vi "CalculateCircle.vi"(5 "Robot":dbl[](array[numeric]), 6 "RealCamera":cluster{"X":dbl, "Y":dbl} {"X" format="%#_13g"}, 7 "Camera":dbl[](array[numeric]), 8 "错误输入（无错误）":errorcluster, 10 "Circle.Steps":dbl[][](array[numeric]), 11 "Circle.Points":dbl[][](array[numeric])) -> (0 "错误输出":errorcluster, 2 "RobotY":dbl, 3 "RobotX":dbl)   [LabVIEW 2016]
uses:
  X86/halcondotnet.dll
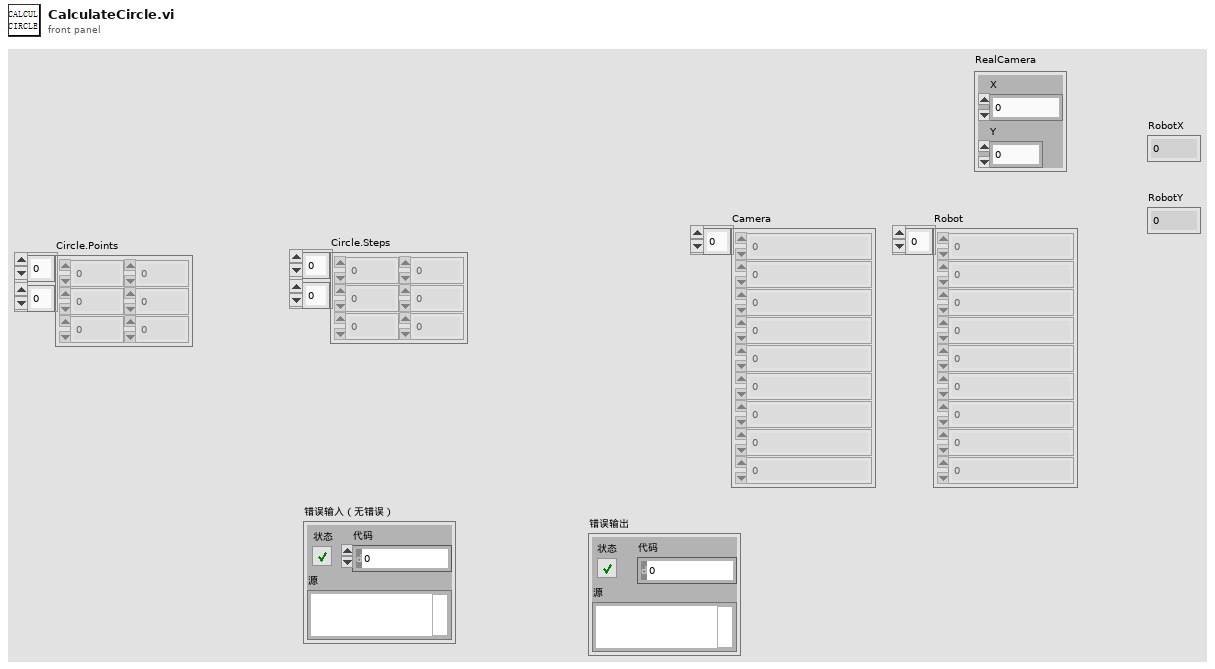
[diagram p1: front panel]
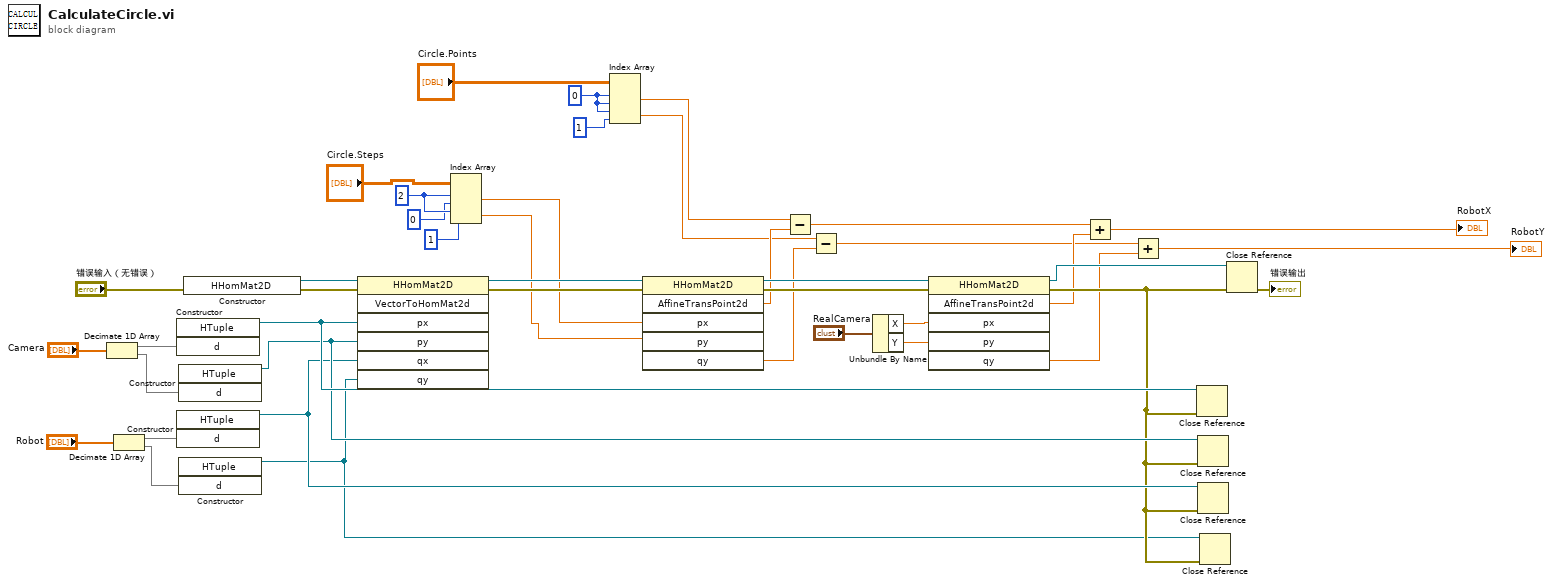
[diagram p0: block diagram]
diagram:
  w4 = 0 ("索引 (行)")
  w11 = 2 ("索引 (行)")
  n1 = Decimate 1D Array("Camera") -> (w40:dbl[], w39:dbl[])
  n2 = Decimate 1D Array("Robot") -> (w38:dbl[], w37:dbl[])
  n3 = constructor class="HTuple"("d"=w40) -> (reference out=w30:refnum<k24>)  [unwired: 3 in, 3 out]
  n4 = constructor class="HTuple"("d"=w38) -> (reference out=w28:refnum<k24>)  [unwired: 3 in, 3 out]
  n5 = constructor class="HTuple"("d"=w39) -> (reference out=w29:refnum<k24>)  [unwired: 3 in, 3 out]
  n6 = constructor class="HTuple"("d"=w37) -> (reference out=w26:refnum<k24>)  [unwired: 3 in, 3 out]
  n7 = constructor class="HHomMat2D"(error in="错误输入（无错误）") -> (reference out=w42:refnum<k24>, error out=w34:errorcluster)  [unwired: 2 in, 1 out]
  n8 = invoke class="HHomMat2D" method="VectorToHomMat2d"(reference=w42, error in=w34, "px"=w30, "py"=w29, "qx"=w28, "qy"=w26) -> (reference out=w41:refnum<k24>, error out=w33:errorcluster)  [unwired: 1 in, 5 out]
  n9 = Index Array(array="Circle.Steps", index (row) #1=w11, index (col) #1=0 ("索引 (行)"), index (row) #2=w11, index (col) #2=1 ("索引 (行)")) -> (element #1=w7:dbl, element #2=w6:dbl)
  n10 = Index Array(array="Circle.Points", index (row) #1=w4, index (col) #1=w4, index (row) #2=w4, index (col) #2=1 ("索引 (行)")) -> (element #1=w2:dbl, element #2=w1:dbl)
  n11 = invoke class="HHomMat2D" method="AffineTransPoint2d"(reference=w41, error in=w33, "px"=w7, "py"=w6) -> (reference out=w35:refnum<k24>, error out=w32:errorcluster, "AffineTransPoint2d"=w20:dbl, "qy"=w19:dbl)  [unwired: 2 in, 2 out]
  n12 = Subtract(x=w2, y=w20) -> (x-y=w16:dbl)
  n13 = Subtract(x=w1, y=w19) -> (x-y=w15:dbl)
  n14 = Unbundle By Name("RealCamera") -> ("X"=w23:dbl, "Y"=w22:dbl)
  n15 = invoke class="HHomMat2D" method="AffineTransPoint2d"(reference=w35, error in=w32, "px"=w23, "py"=w22) -> (reference out=w31:refnum<k24>, error out=w27:errorcluster, "AffineTransPoint2d"=w18:dbl, "qy"=w17:dbl)  [unwired: 2 in, 2 out]
  n16 = Add(x=w16, y=w18) -> (x+y=→"RobotX":dbl)
  n17 = Add(x=w15, y=w17) -> (x+y=→"RobotY":dbl)
  n18 = Close Reference(reference=w30, error in (no error)=w27) -> ()  [unwired: 1 out]
  n19 = Close Reference(reference=w29, error in (no error)=w27) -> ()  [unwired: 1 out]
  n20 = Close Reference(reference=w28, error in (no error)=w27) -> ()  [unwired: 1 out]
  n21 = Close Reference(reference=w26, error in (no error)=w27) -> ()  [unwired: 1 out]
  n22 = Close Reference(reference=w31, error in (no error)=w27) -> (error out=→"错误输出":errorcluster)
